vi "PH_Beamline_Common.set Rotation Stage.vi"(2 "CtlRef":refnum<vi>, 4 "GUI Instance does not exist or here?":bool, 5 "error in (no error)":errorcluster) -> (19 "error out":errorcluster)   [LabVIEW 2014, in "PH_Beamline_Common.lvlib"]
uses:
  PH_Beamline_Common.lvlib
  PH_Common/PH_Common.lvlib
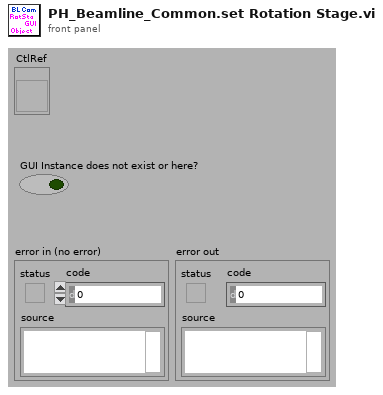
[diagram p1: front panel]
types:
  T1 = cluster{"left":i16, "top":i16, "right":i16, "bottom":i16}
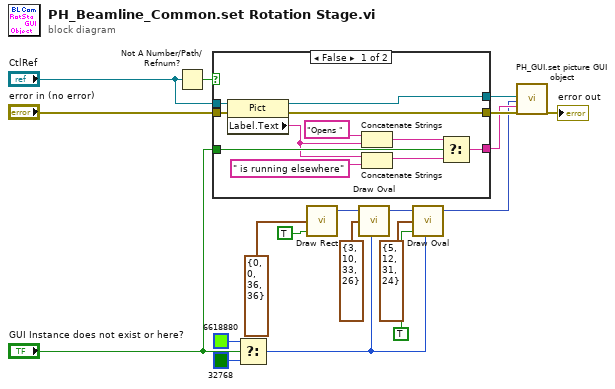
[diagram p0: block diagram]
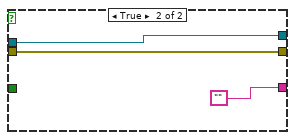
[diagram p2: hidden frame]
diagram:
  n1 = Not A Number/Path/Refnum?(number/path/refnum="CtlRef") -> (NaN/Path/Refnum?=w16:bool)
  n2 = case shown="False" w16 {
    tunnel: "CtlRef" -> [w29 w33]
    tunnel: "error in (no error)" -> [w28 w32]
    tunnel: [w27 w33] -> w12
    tunnel: [w26 w32] -> w14
    tunnel: [w22 ""] -> w11
    tunnel: "GUI Instance does not exist or here?" -> [w21 _]
    frame False {
      n3 = property class="Pict"(reference=w29, error in=w28) -> (reference out=w27:refnum<vi>, error out=w26:errorcluster, "Label.Text"=w20:string)
      n4 = Concatenate Strings("Opens " ("string"), w20) -> (w23:string)
      n5 = Concatenate Strings(w20, " is running elsewhere" ("string")) -> (w24:string)
      n6 = Select(t=w23, s=w21, f=w24) -> (s? t:f=w22:string)
    }
    frame True {
    }
  }
  n7 = Select(t=u32 6618880, s="GUI Instance does not exist or here?", f=u32 32768 ("Color Box")) -> (s? t:f=w4:u32)
  n8 = call <vilib>:"Draw Rect.vi"("rect"=T1 {"left"=0, "top"=0, "right"=36, "bottom"=36}, "fill?(F)"=TRUE) -> ("new picture"=w7:picture)  [unwired: 7 in]
  n9 = call <vilib>:"Draw Oval.vi"("picture"=w7, "rect"=T1 {"left"=3, "top"=10, "right"=33, "bottom"=26}, "color(black)"=w4) -> ("new picture"=w6:picture)  [unwired: 6 in]
  n10 = call <vilib>:"Draw Oval.vi"("picture"=w6, "rect"=T1 {"left"=5, "top"=12, "right"=31, "bottom"=24}, "fill?(F)"=TRUE, "color(black)"=w4) -> ("new picture"=w5:picture)  [unwired: 5 in]
  n11 = call "PH_GUI.set picture GUI object.vi"("CtlRef"=w12, "Picture"=w5, "Tip Strip (\"\")"=w11, "error in (no error)"=w14) -> ("error out"=→"error out":errorcluster)  [unwired: 15 in]
